vi "CRYHardware Editor.vi"() -> ()   [LabVIEW 2013]
uses:
  <vilib>/Utility/miscctls.llb/LVBoundsTypeDef.ctl
  Typedef Control/CRY6175Hardware.ctl
  CRYProject/CRYProject Editor Global.vi
  CRYWindow/SubVI/CRYMain Sub Window Global.vi
  CRYHardware Global.vi
  CRYMainGlobal.vi
  Calibration/SubVI/CRYCal Global.vi
panel:
  out "Proper VI No 2":i32 caption="Proper VI No"
  out "Hardware# Bk":T1
  in  "IN_Channel 1 Old":u16(ring) caption="Channel" items=["Mic 3/4", "Imp 1 L/R", "Imp 1 L/R Single-end", "Imp 2 L/R", "Imp 3 L/R", "Imp 4 L/R", "DUT Mic L/R", "DUT Mic DC L/R", "Cal L/R", "Input 3/4", "Output 1/2", "Output 1(-20dB)"]
  out "Hardware#":T1
  out "EndFlag":bool
  in  "AddStep":bool
  out "StepName":string
  in  "Load Test":bool caption="Load"
  out "VIMiniumBound":T2
  out "Proper VI No":i32
  in  "Board Tab":enum32{"Page 1", "Page 2"}(tab)
  in  "Cancel":bool caption="Apply"
  in  "OK":bool caption="Apply"
  in  "Main Tab":enum32{"Setting", "Help"}(tab)
  out "Microphone":bool caption="咪头"
  in  "Mic Apply":bool caption="Apply"
  in  "OUT_Impedance 2":i32(ring) caption="耳机阻抗 B" items=["1", "33"]
  in  "Mic Resis":i32 caption="咪头电阻" min=-9999 max=99999
  in  "Mic Volt":i32 caption="咪头电压" min=-999 max=9999
  in  "OUT_Impedance 1":i32(ring) caption="耳机阻抗 A" items=["1", "33 差分", "33 单端", "150", "600", "750"]
  in  "IN_Channel 2":u16(ring) caption="端口" items=["传声器 1/2", "传声器 3/4", "传声器 5/6", "传声器 7/8", "线路输入 L/R", "咪头 L/R", "耳机阻抗 B L/R", "内部校准信号 L/R"]
  out "Output":bool caption="声卡输出 1/2"
  in  "IN_Gain 2":i32(ring) caption="放大" items=["-20", "-10", "0", "10", "20", "30", "40", "50"]
  in  "OUT_Channel":u16(ring) caption="端口" items=["仿真嘴 1", "仿真嘴 2", "耳机 A/B", "耳机 A/B(L=R)"]
  out "Input 2":bool caption="声卡输入 3/4"
  in  "IN_Gain 1":i32(ring) caption="放大" items=["-20", "-10", "0", "10", "20", "30"]
  in  "IN_Channel 1":u16(ring) caption="端口" items=["传声器 3/4", "耳机阻抗 A L/R", "耳机阻抗 B L/R", "耳机阻抗 C L/R", "耳机阻抗 D L/R", "咪头电流 L/R", "咪头电压 L/R", "内部校准信号 L/R", "声卡输入 3/4", "声卡输出 1/2", "声卡输出 1(-20dB)"]
  out "Input 1":bool caption="声卡输入 1/2"
  in  "Help":string
  in  "Apply":bool
  in  "Revert":bool caption="Apply"
  in  "Save As...":bool caption="Apply"
  in  "Load...":bool caption="Apply"
  in  "stop":bool
  in  "Channel":i32=1
  in  "Hardware in":string
  in  "Calibration in":string
  # "dB"
  # "Ohm"
  # "dB"
  # "Ohm"
  # "mV"
  # "Ohm"
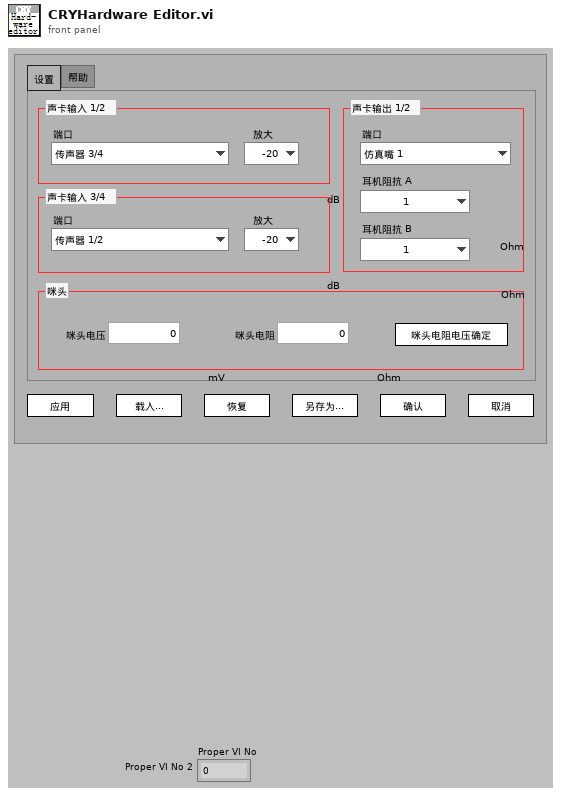
[diagram p1: front panel]
types:
  T1 = typedef "CRY6175Hardware.ctl" = cluster{"Tab Value":u16, "Help":string, "In Channel 1":u16, "In Channel 2":u16, "In Gain 1":i32, "In Gain 2":i32, "Mic Volt":i32, "Mic Resis":i32, "Out Channel":u16, "OUT_Impedance 1":u16, "OUT_Impedance 2":u16, "IN_Channel 1 Old":u16}
  T2 = typedef "LVBoundsTypeDef.ctl" = cluster{"Width":u32, "Height":u32}
  T3 = typedef "CRYStep.ctl" = cluster{"No.VI":i32, "Category":string, "StepName":string, "Seq setup flattened":string, "Comment":string, "Steps config.":bool[], "Jump config":i32[], "Start":dbl, "Increment":dbl, "Name":string, "Unit":string, "Y data":u16, "Y prefix":string, "Y dB ref":dbl, "Y unit":string, "Repeat State Array":cluster{"Start":dbl, "Increment":dbl, "Count":i32, "Num":i32}[]}
  T4 = enum16{"OK", "Yes", "YesNo", "YesNoCancel", "ReplaceAppend"}
  T5 = cluster{"Load Test":bool, "Apply":bool, "Mic Apply":bool, "OK":bool, "Cancel":bool}
  T6 = typedef "CRYData Cluster Array.ctl" = T7[]
  T7 = typedef "CRYData Cluster.ctl" = cluster{"Name":string, "Curve":cluster{"x":dbl, "y":dbl, "z":dbl}[], "X data":u16, "Y data":u16, "Z data":u16, "X axis":u16, "Y axis":u16, "Z axis":u16, "X unit":string, "Y unit":string, "Z unit":string, "X dB ref":dbl, "Y dB ref":dbl, "Z dB ref":dbl, "single val":bool, "protected":bool, "display X":bool, "display Y":bool, "display Z":bool, "Test Info":string, "Step No.":i32, "Plot Settings":cluster{"Color":u32, "Interpolation":u8, "Point Style":u8, "Line Style":u8, "Point Color":u32, "Line Width":u8, "Bar Plot Style":u8, "Fill To":i16}, "AutoProtect":bool}
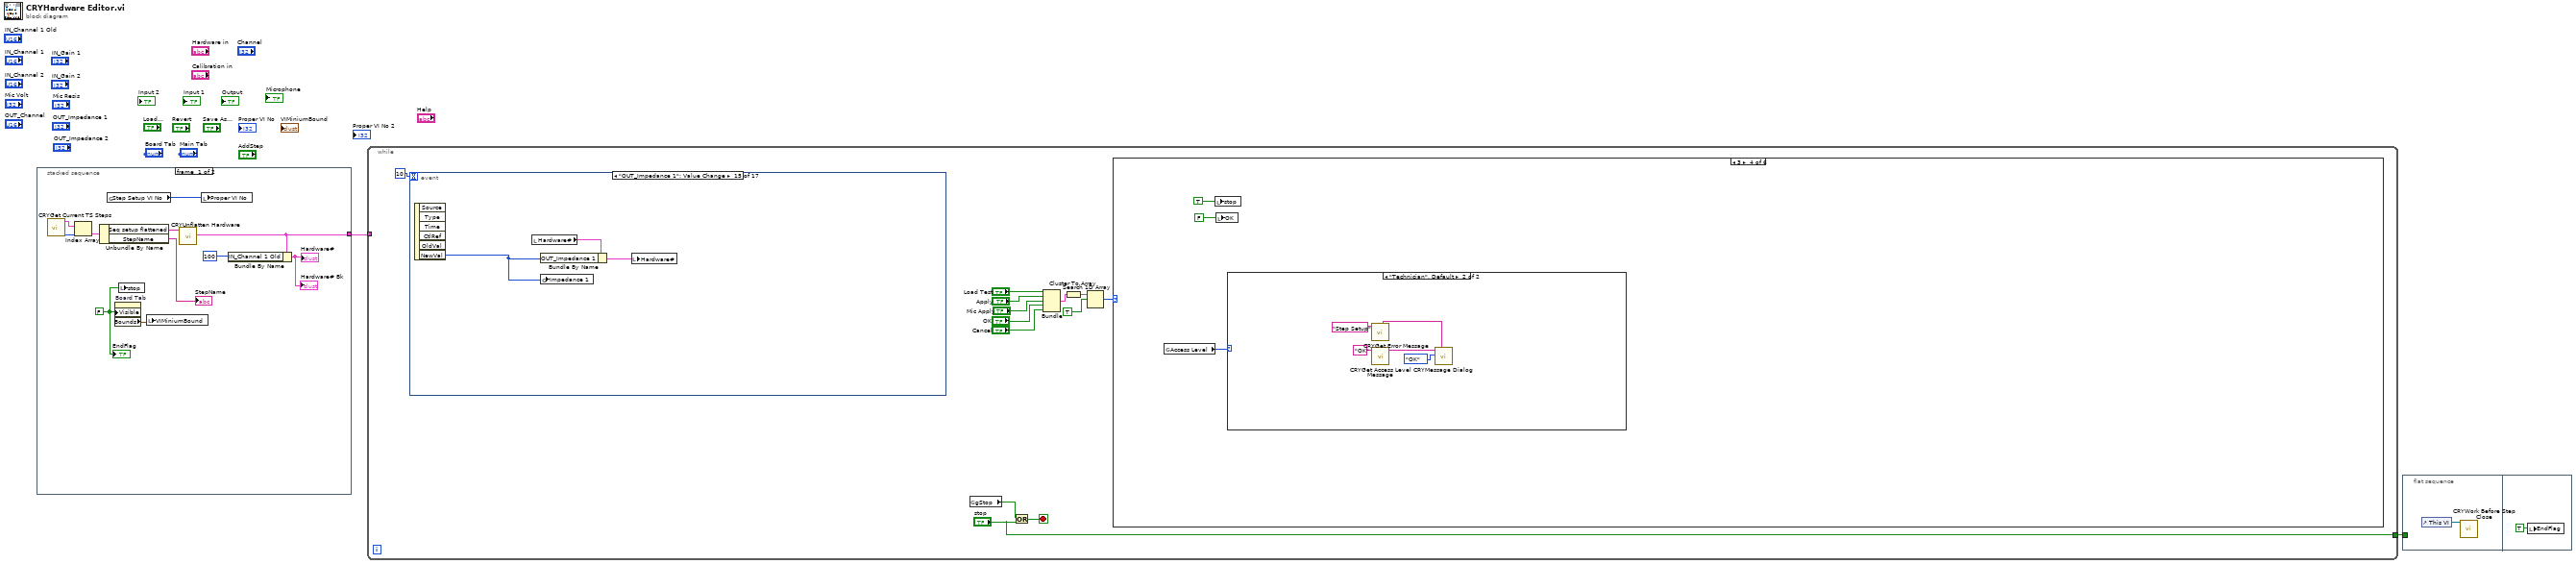
[diagram p0: block diagram]
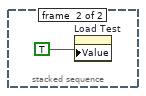
[diagram p2: hidden frame]
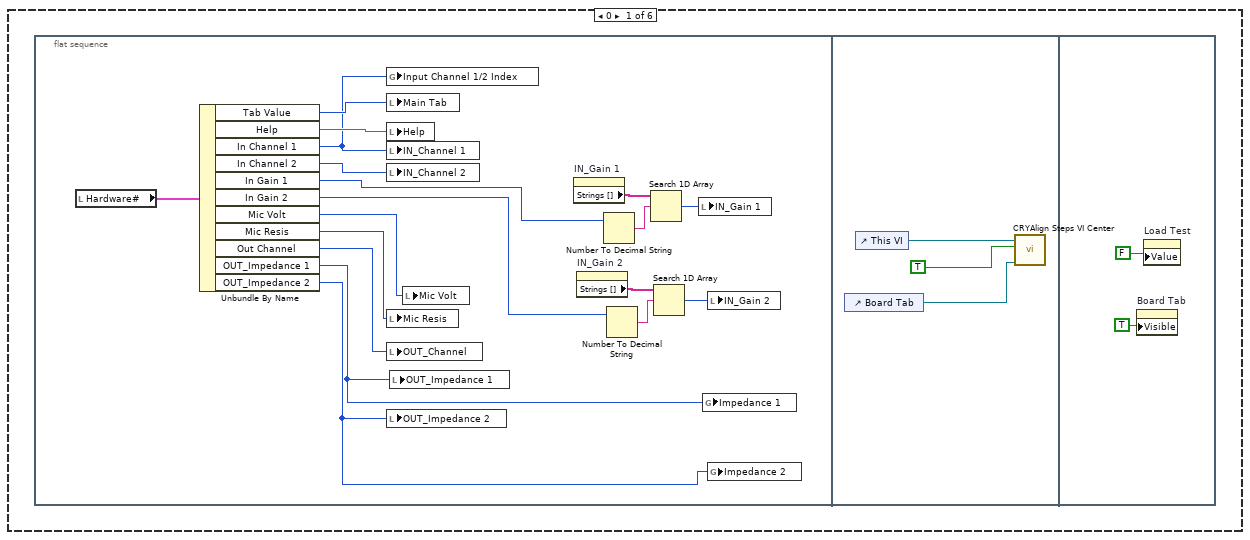
[diagram p3: hidden frame]
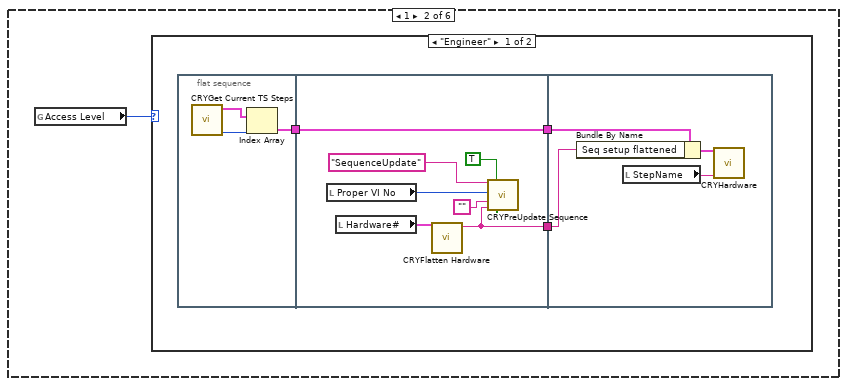
[diagram p4: hidden frame]
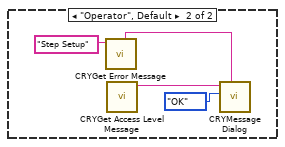
[diagram p5: hidden frame]
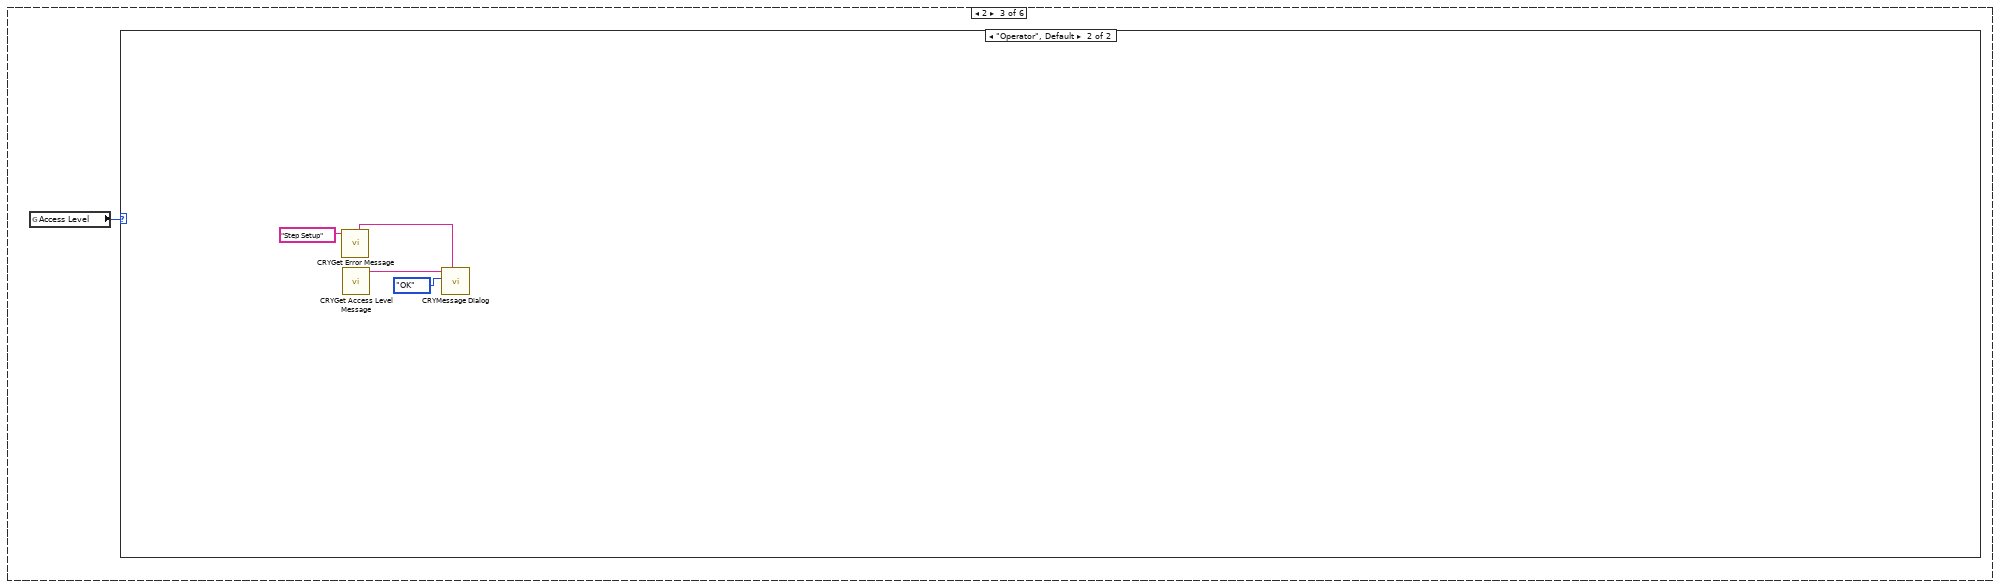
[diagram p6: hidden frame]
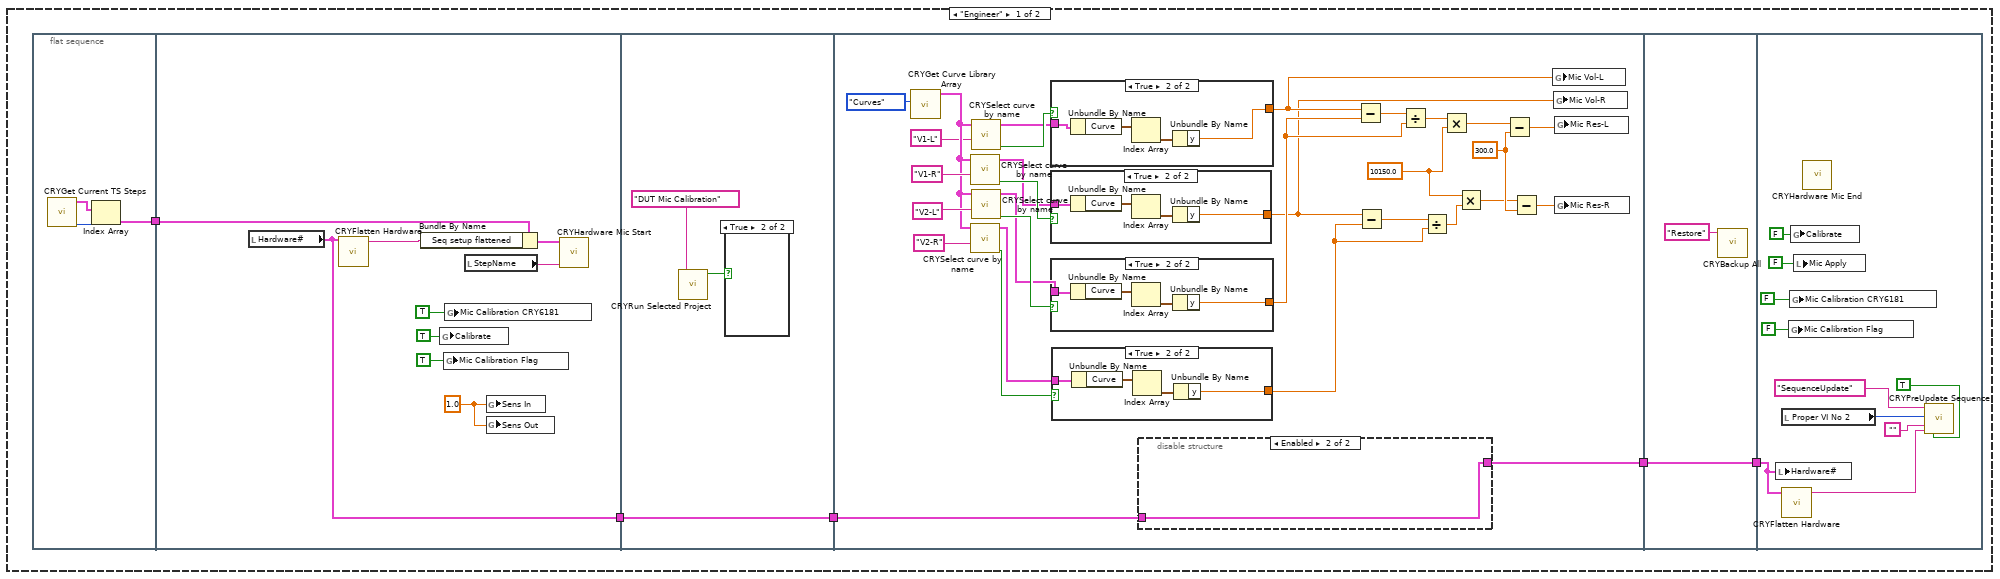
[diagram p7: hidden frame]
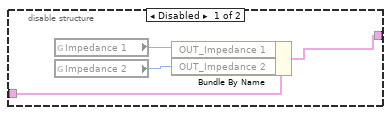
[diagram p9: hidden frame]
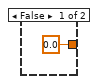
[diagram p10: hidden frame]
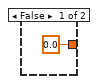
[diagram p11: hidden frame]
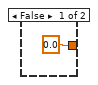
[diagram p12: hidden frame]
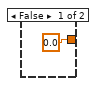
[diagram p13: hidden frame]
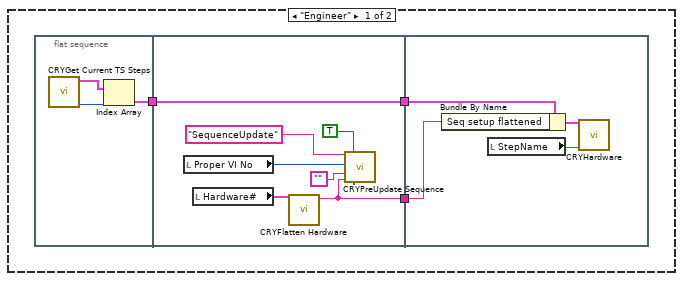
[diagram p14: hidden frame]
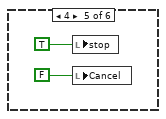
[diagram p15: hidden frame]
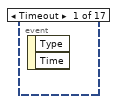
[diagram p17: hidden frame]
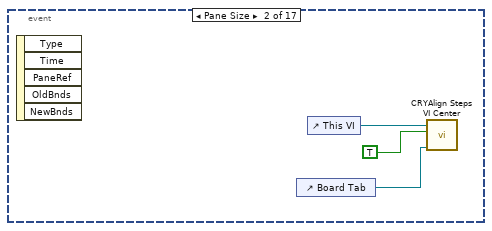
[diagram p18: hidden frame]
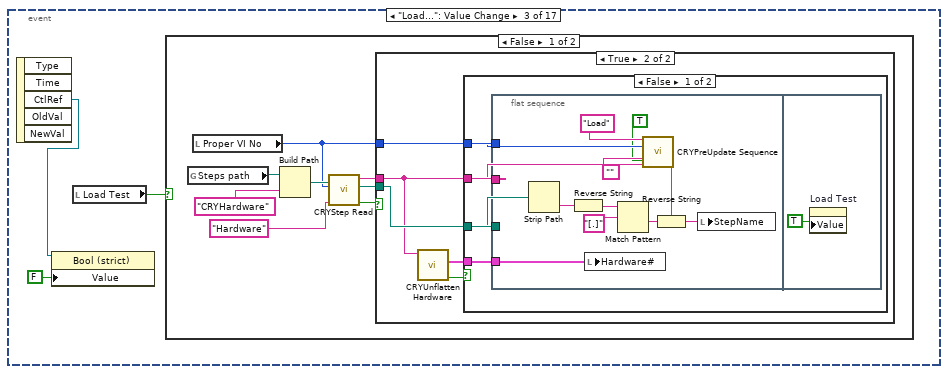
[diagram p19: hidden frame]
diagram:
  n1 = stacked-sequence {
    tunnel: [w5 _] -> w1
    frame #0 {
      w3 = FALSE ("Visible")
      n2 = call "CRYGet Current TS Steps.vi"() -> ("SelectStepNumber in Tree"=w11:i32, "Steps"=w12:T3[])  [unwired: 7 in, 3 out]
      n3 = Index Array(array=w12, index=w11) -> (element=w13:T3)
      n4 = Unbundle By Name(w13) -> ("Seq setup flattened"=w8:string, "StepName"=→"StepName":string)
      n5 = global read "CRYProject Editor Global.vi" "Step Setup VI No"() -> (w10:i32)
      n6 = property on="Board Tab" class="TabCtl (strict)"("Visible"=w3) -> ("Bounds"=w9:T2)  [unwired: 2 in, 2 out]
      n7 = local write "stop"(w3) -> ()
      n8 = local write "VIMiniumBound"(w9) -> ()
      n9 = call "CRYUnflatten Hardware.vi"("Unflatten Hardware#"=w8) -> ("Hardware"=w5:T1)  [unwired: 8 in, 2 out]
      n10 = local write "Proper VI No"(w10) -> ()
      n11 = Bundle By Name(cluster=w5, "IN_Channel 1 Old"=u16 100) -> (→"Hardware#" →"Hardware# Bk":T1)
      "EndFlag" <- w3
    }
    frame #1 {
      n12 = property on="Load Test" class="Bool (strict)"("Value"=TRUE ("Load Test")) -> ()  [unwired: 2 in, 2 out]
    }
  }
  n13 = while {
    tunnel: ["stop"] -> w2
    tunnel: w1 -> [_]
    stop <- w25 stop-if-true
    n14 = event shown="[14] \"OUT_Impedance 1\": Value Change" {
      selector: _ -> [_ _ _ _ _ _ _ _ _ _ _ _ _ _ _ _ _]
      dyn-events: _ -> [_ _ _ _ _ _ _ _ _ _ _ _ _ _ _ _ _]
      timeout: 10 -> [_ _ _ _ _ _ _ _ _ _ _ _ _ _ _ _ _]
      event Timeout {
        n15 = event-data() -> ()  [unwired: 1 in, 2 out]
      }
      event Pane Size {
        n16 = event-data() -> ()  [unwired: 1 in, 5 out]
        n17 = control-ref of="Board Tab"() -> (w192:refnum<vi>)
        n18 = control-ref of="This VI"() -> (w194:refnum<vi>)
        n19 = call "CRYAlign Steps VI Center.vi"("Tab2"=w192, "Input/Output"=TRUE, "VIRef"=w194) -> ()  [unwired: 1 in, 8 out]
      }
      event "Load...": Value Change {
        n20 = event-data() -> ("CtlRef"=w195:refnum<vi>)  [unwired: 1 in, 4 out]
        n21 = property class="Bool (strict)"(reference=w195, "Value"=FALSE) -> ()  [unwired: 1 in, 2 out]
        n22 = local read "Load Test"() -> (w197:bool)
        n23 = case shown="False" w197 {
          frame False {
            n24 = global read "CRYMainGlobal.vi" "Steps path"() -> (w204:path)
            n25 = local read "Proper VI No"() -> (w198:i32)
            n26 = Build Path(base path=w204, name or relative path="CRYHardware") -> (appended path=w205:path)
            n27 = call "CRYStep Read.vi"("Category Name"="Hardware" ("Step File Name"), "Proper VI No"=w198, "Step File Path"=w205) -> ("status"=w201:bool, "selected path"=w199:path, "Flatten Step"=w200:string)  [unwired: 1 in, 3 out]
            n28 = case shown="True" w201 {
              tunnel: w200 -> [_ w207]
              tunnel: w199 -> [_ w208]
              tunnel: w198 -> [_ w206]
              frame False {
              }
              frame True {
                n29 = call "CRYUnflatten Hardware.vi"("Unflatten Hardware#"=w207) -> ("Error?"=w210:bool, "Hardware"=w209:T1)  [unwired: 8 in, 1 out]
                n30 = case shown="False" w210 {
                  tunnel: w209 -> [w214 _]
                  tunnel: w208 -> [w213 _]
                  tunnel: w207 -> [w212 _]
                  tunnel: w206 -> [w211 _]
                  frame False {
                    n31 = flat-sequence {
                      tunnel: w214 -> [w226]
                      tunnel: w213 -> [w223]
                      tunnel: w212 -> [w222]
                      tunnel: w211 -> [w221]
                      frame #0 {
                        n32 = Strip Path(path=w223) -> (name=w216:string)  [unwired: 1 out]
                        n33 = Reverse String(1:w216) -> (0:w218:string)
                        n34 = local write "Hardware#"(w226) -> ()
                        n35 = Match Pattern(string=w218, regular expression="[.]") -> (after substring=w219:string)  [unwired: 4 out]
                        n36 = Reverse String(1:w219) -> (0:w215:string)
                        n37 = call "CRYPreUpdate Sequence.vi"("EventName"="Load", "StepName Arg3"=w215, "Proper VI No"=w221, "Project View Step Name Identifier Arg1"="", "Step flattened Arg2"=w222, "AllChangeFlg"=TRUE ("Name/Identifier")) -> ()  [unwired: 10 in]
                        n38 = local write "StepName"(w215) -> ()
                      }
                      frame #1 {
                        n39 = property on="Load Test" class="Bool (strict)"("Value"=TRUE ("Load Test")) -> ()  [unwired: 2 in, 2 out]
                      }
                    }
                  }
                  frame True {
                  }
                }
              }
            }
          }
          frame True {
          }
        }
      }
      event "Save As...": Value Change {
        w236 = "Hardware" ("Step File Name")
        n40 = event-data() -> ("CtlRef"=w228:refnum<vi>)  [unwired: 1 in, 4 out]
        n41 = local read "Hardware#"() -> (w231:T1)
        n42 = property class="Bool (strict)"(reference=w228, "Value"=FALSE) -> ()  [unwired: 1 in, 2 out]
        n43 = global read "CRYMainGlobal.vi" "Steps path"() -> (w242:path)
        n44 = call "CRYFlatten Hardware.vi"("Hardware#"=w231) -> ("Hardware# flattened"=w235:string)  [unwired: 10 in]
        n45 = Build Path(base path=w242, name or relative path="CRYHardware") -> (appended path=w238:path)
        n46 = local read "Proper VI No"() -> (w237:i32)
        n47 = call "CRYStep Write.vi"("StepIdentifier"="", "Default"=FALSE, "Proper VI No"=w237, "Category Name"=w236, "Step File Path"=w238, "Step flattened"=w235, "Step File Name"=w236) -> ("name"=w233:string, "Cancel"=w234:bool)  [unwired: 1 in, 2 out]
        n48 = Match Pattern(string=w233, regular expression=".har") -> (before substring=w230:string)  [unwired: 1 in, 3 out]
        n49 = case shown="False" w234 {
          tunnel: w230 -> [w243 _]
          frame False {
            n50 = Current VI's Path() -> (path=w244:path)
            n51 = call "CRYTitle bar update.vi"("Step name"=w243, "Editor VI path"=w244) -> ()  [unwired: 10 in]
          }
          frame True {
          }
        }
      }
      event "Revert": Value Change {
        n52 = event-data() -> ("CtlRef"=w246:refnum<vi>)  [unwired: 1 in, 4 out]
        n53 = flat-sequence {
          frame #0 {
            n54 = local read "Hardware# Bk"() -> (w247:T1)
            n55 = local write "Hardware#"(w247) -> ()
          }
          frame #1 {
            n56 = property on="Load Test" class="Bool (strict)"("Value"=TRUE ("Load Test")) -> ()  [unwired: 2 in, 2 out]
          }
        }
        n57 = property class="Bool (strict)"(reference=w246, "Value"=FALSE) -> ()  [unwired: 1 in, 2 out]
      }
      event Panel Close {
        n58 = event-data() -> ()  [unwired: 1 in, 4 out]
        n59 = control-ref of="This VI"() -> (w250:refnum<vi>)
        n60 = local write "Cancel"(TRUE ("Cancel")) -> ()
        n61 = call "CRYWork Before Step Close.vi"("StepVI Ref"=w250) -> ()  [unwired: 11 in]
      }
      event "Main Tab": Value Change {
        n62 = event-data() -> ("NewVal"=w252:enum32{"Setting", "Help"})  [unwired: 1 in, 4 out]
        n63 = local read "Hardware#"() -> (w253:T1)
        n64 = Bundle By Name(cluster=w253, "Tab Value"=w252) -> (w251:T1)
        n65 = local write "Hardware#"(w251) -> ()
      }
      event "IN_Channel 1": Value Change {
        n66 = event-data() -> ("OldVal"=w255:u16, "NewVal"=w254:u16)  [unwired: 1 in, 4 out]
        n67 = local read "Hardware#"() -> (w257:T1)
        n68 = local write "IN_Channel 1 Old"(w255) -> ()
        n69 = Bundle By Name(cluster=w257, "In Channel 1"=w254) -> (w256:T1)
        n70 = global write "CRYHardware Global.vi" "Input Channel 1/2 Index"(w254) -> ()
        n71 = local write "Hardware#"(w256) -> ()
      }
      event "IN_Gain 1": Value Change {
        n72 = event-data() -> ("NewVal"=w259:i32)  [unwired: 1 in, 5 out]
        n73 = property on="IN_Gain 1" class="Ring (strict)"() -> ("Strings []"=w261:string[])  [unwired: 2 in, 2 out]
        n74 = Index Array(array=w261, index=w259) -> (element=w260:string)
        n75 = Decimal String To Number(string=w260) -> (number=w258:i32)  [unwired: 2 in, 1 out]
        n76 = local read "Hardware#"() -> (w263:T1)
        n77 = Bundle By Name(cluster=w263, "In Gain 1"=w258) -> (w262:T1)
        n78 = local write "Hardware#"(w262) -> ()
      }
      event "IN_Channel 2": Value Change {
        n79 = event-data() -> ("NewVal"=w264:u16)  [unwired: 1 in, 5 out]
        n80 = local read "Hardware#"() -> (w266:T1)
        n81 = Bundle By Name(cluster=w266, "In Channel 2"=w264) -> (w265:T1)
        n82 = local write "Hardware#"(w265) -> ()
      }
      event "IN_Gain 2": Value Change {
        n83 = event-data() -> ("NewVal"=w268:i32)  [unwired: 1 in, 5 out]
        n84 = property on="IN_Gain 2" class="Ring (strict)"() -> ("Strings []"=w269:string[])  [unwired: 2 in, 2 out]
        n85 = Index Array(array=w269, index=w268) -> (element=w270:string)
        n86 = Decimal String To Number(string=w270) -> (number=w267:i32)  [unwired: 2 in, 1 out]
        n87 = local read "Hardware#"() -> (w272:T1)
        n88 = Bundle By Name(cluster=w272, "In Gain 2"=w267) -> (w271:T1)
        n89 = local write "Hardware#"(w271) -> ()
      }
      event "Mic Volt": Value Change {
        n90 = event-data() -> ("NewVal"=w273:i32)  [unwired: 1 in, 5 out]
        n91 = local read "Hardware#"() -> (w275:T1)
        n92 = Bundle By Name(cluster=w275, "Mic Volt"=w273) -> (w274:T1)
        n93 = local write "Hardware#"(w274) -> ()
      }
      event "Mic Resis": Value Change {
        n94 = event-data() -> ("NewVal"=w276:i32)  [unwired: 1 in, 5 out]
        n95 = local read "Hardware#"() -> (w278:T1)
        n96 = Bundle By Name(cluster=w278, "Mic Resis"=w276) -> (w277:T1)
        n97 = local write "Hardware#"(w277) -> ()
      }
      event "OUT_Channel": Value Change {
        n98 = event-data() -> ("NewVal"=w279:u16)  [unwired: 1 in, 5 out]
        n99 = local read "Hardware#"() -> (w281:T1)
        n100 = Bundle By Name(cluster=w281, "Out Channel"=w279) -> (w280:T1)
        n101 = local write "Hardware#"(w280) -> ()
      }
      event "OUT_Impedance 1": Value Change {
        n102 = event-data() -> ("NewVal"=w282:i32)  [unwired: 1 in, 5 out]
        n103 = local read "Hardware#"() -> (w284:T1)
        n104 = Bundle By Name(cluster=w284, "OUT_Impedance 1"=w282) -> (w283:T1)
        n105 = global write "CRYHardware Global.vi" "Impedance 1"(w282) -> ()
        n106 = local write "Hardware#"(w283) -> ()
      }
      event "OUT_Impedance 2": Value Change {
        n107 = event-data() -> ("NewVal"=w285:i32)  [unwired: 1 in, 5 out]
        n108 = local read "Hardware#"() -> (w287:T1)
        n109 = global write "CRYHardware Global.vi" "Impedance 2"(w285) -> ()
        n110 = Bundle By Name(cluster=w287, "OUT_Impedance 2"=w285) -> (w286:T1)
        n111 = local write "Hardware#"(w286) -> ()
      }
      event "Help": Value Change {
        n112 = event-data() -> ("NewVal"=w289:string)  [unwired: 1 in, 4 out]
        n113 = local read "Hardware#"() -> (w290:T1)
        n114 = Bundle By Name(cluster=w290, "Help"=w289) -> (w288:T1)
        n115 = local write "Hardware#"(w288) -> ()
      }
    }
    n116 = global read "CRYMain Sub Window Global.vi" "gStop"() -> (w26:bool)
    n117 = Or(x=w26, y="stop") -> (x .or. y?=w25:bool)
    n118 = Bundle("Load Test"="Load Test", "Apply"="Apply", "Mic Apply"="Mic Apply", "OK"="OK", "Cancel"="Cancel") -> (w24:T5)  [unwired: 1 out]
    n119 = Cluster To Array(cluster=w24) -> (array=w23:bool[])
    n120 = Search 1D Array(1D array=w23, element=TRUE) -> (index of element=w20:i32)  [unwired: 1 out]
    n121 = case shown="3" w20 {
      frame 0 {
        n122 = flat-sequence {
          frame #0 {
            n123 = local read "Hardware#"() -> (w45:T1)
            n124 = Unbundle By Name(w45) -> ("Tab Value"=w44:u16, "Help"=w43:string, "In Channel 1"=w29:u16, "In Channel 2"=w42:u16, "In Gain 1"=w39:i32, "In Gain 2"=w33:i32, "Mic Volt"=w41:i32, "Mic Resis"=w31:i32, "Out Channel"=w40:u16, "OUT_Impedance 1"=w30:u16, "OUT_Impedance 2"=w28:u16)
            n125 = global write "CRYHardware Global.vi" "Input Channel 1/2 Index"(w29) -> ()
            n126 = local write "Main Tab"(w44) -> ()
            n127 = local write "Help"(w43) -> ()
            n128 = local write "IN_Channel 1"(w29) -> ()
            n129 = local write "IN_Channel 2"(w42) -> ()
            n130 = local write "Mic Resis"(w31) -> ()
            n131 = local write "OUT_Channel"(w40) -> ()
            n132 = local write "OUT_Impedance 2"(w28) -> ()
            n133 = local write "OUT_Impedance 1"(w30) -> ()
            n134 = local write "Mic Volt"(w41) -> ()
            n135 = property on="IN_Gain 1" class="Ring (strict)"() -> ("Strings []"=w37:string[])  [unwired: 2 in, 2 out]
            n136 = property on="IN_Gain 2" class="Ring (strict)"() -> ("Strings []"=w35:string[])  [unwired: 2 in, 2 out]
            n137 = Number To Decimal String(number=w39) -> (decimal integer string=w38:string)  [unwired: 1 in]
            n138 = Number To Decimal String(number=w33) -> (decimal integer string=w34:string)  [unwired: 1 in]
            n139 = Search 1D Array(1D array=w37, element=w38) -> (index of element=w36:i32)  [unwired: 1 in]
            n140 = Search 1D Array(1D array=w35, element=w34) -> (index of element=w32:i32)  [unwired: 1 in]
            n141 = local write "IN_Gain 1"(w36) -> ()
            n142 = global write "CRYHardware Global.vi" "Impedance 1"(w30) -> ()
            n143 = local write "IN_Gain 2"(w32) -> ()
            n144 = global write "CRYHardware Global.vi" "Impedance 2"(w28) -> ()
          }
          frame #1 {
            n145 = control-ref of="Board Tab"() -> (w46:refnum<vi>)
            n146 = control-ref of="This VI"() -> (w48:refnum<vi>)
            n147 = call "CRYAlign Steps VI Center.vi"("Tab2"=w46, "Input/Output"=TRUE, "VIRef"=w48) -> ()  [unwired: 1 in, 8 out]
          }
          frame #2 {
            n148 = property on="Board Tab" class="TabCtl (strict)"("Visible"=TRUE) -> ()  [unwired: 2 in, 2 out]
            n149 = property on="Load Test" class="Bool (strict)"("Value"=FALSE ("Load Test")) -> ()  [unwired: 2 in, 2 out]
          }
        }
      }
      frame 1 {
        n150 = global read "CRYMainGlobal.vi" "Access Level"() -> (w51:enum16{"Engineer", "Technician", "Operator"})
        n151 = case shown="\"Engineer\"" w51 {
          frame "Engineer" {
            n152 = flat-sequence {
              tunnel: [w55] -> w53
              tunnel: [w59] -> w54
              tunnel: w53 -> [w59]
              tunnel: [w58] -> w52
              tunnel: w54 -> [w68]
              tunnel: w52 -> [w67]
              frame #0 {
                n153 = call "CRYGet Current TS Steps.vi"() -> ("SelectStepNumber in Tree"=w56:i32, "Steps"=w57:T3[])  [unwired: 1 in, 9 out]
                n154 = Index Array(array=w57, index=w56) -> (element=w55:T3)
              }
              frame #1 {
                n155 = local read "Proper VI No"() -> (w62:i32)
                n156 = local read "Hardware#"() -> (w60:T1)
                n157 = call "CRYFlatten Hardware.vi"("Hardware#"=w60) -> ("Hardware# flattened"=w58:string)  [unwired: 10 in]
                n158 = call "CRYPreUpdate Sequence.vi"("EventName"="SequenceUpdate", "Proper VI No"=w62, "Project View Step Name Identifier Arg1"="", "Step flattened Arg2"=w58, "AllChangeFlg"=TRUE ("Name/Identifier")) -> ()  [unwired: 11 in]
              }
              frame #2 {
                n159 = Bundle By Name(cluster=w68, "Seq setup flattened"=w67) -> (w66:T3)
                n160 = local read "StepName"() -> (w65:string)
                n161 = call "CRYHardware.vi"("Setup in"=w66, "Step name"=w65) -> ()  [unwired: 9 in, 5 out]
              }
            }
          }
          frame "Operator", Default {
            n162 = call "CRYGet Error Message.vi"("Kind"="Step Setup") -> ("Window Title"=w71:string)  [unwired: 5 in, 5 out]
            n163 = call "CRYGet Access Level Message.vi"() -> ("Multibyte string"=w69:string)  [unwired: 11 in]
            n164 = call "CRYMessage Dialog.vi"("Window Title"=w71, "YesNoCancel"=T4."OK", "Message Content"=w69) -> ()  [unwired: 7 in, 2 out]
          }
        }
      }
      frame 2 {
        n165 = global read "CRYMainGlobal.vi" "Access Level"() -> (w73:enum16{"Engineer", "Technician", "Operator"})
        n166 = case shown="\"Operator\", Default" w73 {
          frame "Engineer" {
            n167 = flat-sequence {
              tunnel: [w79] -> w78
              tunnel: [w82] -> w76
              tunnel: w78 -> [w90]
              tunnel: [w91] -> w77
              tunnel: w76 -> [w91]
              tunnel: w77 -> [w95]
              tunnel: [w94] -> w74
              tunnel: [w149] -> w75
              tunnel: w74 -> [w149]
              tunnel: w75 -> [w156]
              frame #0 {
                n168 = call "CRYGet Current TS Steps.vi"() -> ("SelectStepNumber in Tree"=w80:i32, "Steps"=w81:T3[])  [unwired: 1 in, 9 out]
                n169 = Index Array(array=w81, index=w80) -> (element=w79:T3)
              }
              frame #1 {
                w83 = 1.0 ("Sens In")
                n170 = local read "Hardware#"() -> (w82:T1)
                n171 = call "CRYFlatten Hardware.vi"("Hardware#"=w82) -> ("Hardware# flattened"=w89:string)  [unwired: 10 in]
                n172 = Bundle By Name(cluster=w90, "Seq setup flattened"=w89) -> (w88:T3)
                n173 = global write "CRYCal Global.vi" "Calibrate"(TRUE ("Calibrate")) -> ()
                n174 = global write "CRYHardware Global.vi" "Mic Calibration Flag"(TRUE ("Mic Calibration Flag")) -> ()
                n175 = global write "CRYCal Global.vi" "Mic Calibration CRY6181"(TRUE ("Audio Interface Calibrate")) -> ()
                n176 = local read "StepName"() -> (w87:string)
                n177 = global write "CRYCal Global.vi" "Sens In"(w83) -> ()
                n178 = global write "CRYCal Global.vi" "Sens Out"(w83) -> ()
                n179 = call "CRYHardware Mic Start.vi"("Setup in"=w88, "Step name"=w87) -> ()  [unwired: 9 in, 5 out]
              }
              frame #2 {
                n180 = call "CRYRun Selected Project.vi"("sequence name"="DUT Mic Calibration" ("y")) -> ("run state"=w93:bool)  [unwired: 10 out]
                n181 = case shown="True" w93 {
                  frame False {
                  }
                  frame True {
                  }
                }
              }
              frame #3 {
                w123 = 300.0 ("y")
                w96 = 10150.0 ("y")
                n182 = call "CRYGet Curve Library Array.vi"("Type In"=enum16{"Curves", "Values", "Results", "WFM"}."Curves") -> ("Curve/Value array"=w109:T6)  [unwired: 8 in, 2 out]
                n183 = call "CRYSelect curve by name.vi"("Curve name desired (just name, if flat data not wired)"="V1-R", "Data array"=w109) -> ("Exists?"=w106:bool, "Desired Curve"=w103:T7)  [unwired: 1 in, 7 out]
                n184 = call "CRYSelect curve by name.vi"("Curve name desired (just name, if flat data not wired)"="V2-R", "Data array"=w109) -> ("Exists?"=w108:bool, "Desired Curve"=w105:T7)  [unwired: 1 in, 7 out]
                n185 = call "CRYSelect curve by name.vi"("Curve name desired (just name, if flat data not wired)"="V1-L", "Data array"=w109) -> ("Exists?"=w113:bool, "Desired Curve"=w102:T7)  [unwired: 1 in, 7 out]
                n186 = call "CRYSelect curve by name.vi"("Curve name desired (just name, if flat data not wired)"="V2-L", "Data array"=w109) -> ("Exists?"=w107:bool, "Desired Curve"=w104:T7)  [unwired: 1 in, 7 out]
                n187 = case shown="True" w113 {
                  tunnel: w102 -> [_ w148]
                  tunnel: [0.0 ("y") w145] -> w99
                  frame False {
                  }
                  frame True {
                    n188 = Unbundle By Name(w148) -> ("Curve"=w147:cluster{"x":dbl, "y":dbl, "z":dbl}[])
                    n189 = Index Array(array=w147) -> (element=w146:cluster{"x":dbl, "y":dbl, "z":dbl})  [unwired: 1 in]
                    n190 = Unbundle By Name(w146) -> ("y"=w145:dbl)
                  }
                }
                n191 = case shown="True" w106 {
                  tunnel: w103 -> [_ w143]
                  tunnel: [0.0 ("y") w140] -> w98
                  frame False {
                  }
                  frame True {
                    n192 = Unbundle By Name(w143) -> ("Curve"=w142:cluster{"x":dbl, "y":dbl, "z":dbl}[])
                    n193 = Index Array(array=w142) -> (element=w141:cluster{"x":dbl, "y":dbl, "z":dbl})  [unwired: 1 in]
                    n194 = Unbundle By Name(w141) -> ("y"=w140:dbl)
                  }
                }
                n195 = case shown="True" w107 {
                  tunnel: w104 -> [_ w138]
                  tunnel: [0.0 ("y") w135] -> w115
                  frame False {
                  }
                  frame True {
                    n196 = Unbundle By Name(w138) -> ("Curve"=w137:cluster{"x":dbl, "y":dbl, "z":dbl}[])
                    n197 = Index Array(array=w137) -> (element=w136:cluster{"x":dbl, "y":dbl, "z":dbl})  [unwired: 1 in]
                    n198 = Unbundle By Name(w136) -> ("y"=w135:dbl)
                  }
                }
                n199 = case shown="True" w108 {
                  tunnel: w105 -> [_ w133]
                  tunnel: [0.0 ("y") w130] -> w120
                  frame False {
                  }
                  frame True {
                    n200 = Unbundle By Name(w133) -> ("Curve"=w132:cluster{"x":dbl, "y":dbl, "z":dbl}[])
                    n201 = Index Array(array=w132) -> (element=w131:cluster{"x":dbl, "y":dbl, "z":dbl})  [unwired: 1 in]
                    n202 = Unbundle By Name(w131) -> ("y"=w130:dbl)
                  }
                }
                n203 = disable-structure shown="Enabled" {
                  disable-tunnel: w95 -> [w125 w128]
                  disable-tunnel: [w124 w128] -> w94
                  frame Disabled {
                    n204 = global read "CRYHardware Global.vi" "Impedance 1"() -> (w126:i32)
                    n205 = global read "CRYHardware Global.vi" "Impedance 2"() -> (w127:i32)
                    n206 = Bundle By Name(cluster=w125, "OUT_Impedance 1"=w126, "OUT_Impedance 2"=w127) -> (w124:T1)
                  }
                  frame Enabled {
                  }
                }
                n207 = Subtract(x=w99, y=w115) -> (x-y=w114:dbl)
                n208 = Subtract(x=w98, y=w120) -> (x-y=w119:dbl)
                n209 = Divide(x=w114, y=w115) -> (x/y=w97:dbl)
                n210 = Divide(x=w119, y=w120) -> (x/y=w118:dbl)
                n211 = Multiply(x=w97, y=w96) -> (x*y=w116:dbl)
                n212 = Multiply(x=w96, y=w118) -> (x*y=w117:dbl)
                n213 = Subtract(x=w116, y=w123) -> (x-y=w121:dbl)
                n214 = Subtract(x=w117, y=w123) -> (x-y=w122:dbl)
                n215 = global write "CRYHardware Global.vi" "Mic Vol-L"(w99) -> ()
                n216 = global write "CRYHardware Global.vi" "Mic Vol-R"(w98) -> ()
                n217 = global write "CRYHardware Global.vi" "Mic Res-L"(w121) -> ()
                n218 = global write "CRYHardware Global.vi" "Mic Res-R"(w122) -> ()
              }
              frame #4 {
                n219 = call "CRYBackup All.vi"("sOption"="Restore") -> ()  [unwired: 11 in]
              }
              frame #5 {
                n220 = local write "Hardware#"(w156) -> ()
                n221 = local read "Proper VI No 2"() -> (w155:i32)
                n222 = call "CRYFlatten Hardware.vi"("Hardware#"=w156) -> ("Hardware# flattened"=w151:string)  [unwired: 10 in]
                n223 = global write "CRYHardware Global.vi" "Mic Calibration Flag"(FALSE ("Mic Calibration Flag")) -> ()
                n224 = global write "CRYCal Global.vi" "Mic Calibration CRY6181"(FALSE ("Audio Interface Calibrate")) -> ()
                n225 = global write "CRYCal Global.vi" "Calibrate"(FALSE ("Calibrate")) -> ()
                n226 = local write "Mic Apply"(FALSE ("Mic Apply")) -> ()
                n227 = call "CRYHardware Mic End.vi"() -> ()  [unwired: 16 in]
                n228 = call "CRYPreUpdate Sequence.vi"("EventName"="SequenceUpdate", "Proper VI No"=w155, "Project View Step Name Identifier Arg1"="", "Step flattened Arg2"=w151, "AllChangeFlg"=TRUE ("Name/Identifier")) -> ()  [unwired: 11 in]
              }
            }
          }
          frame "Operator", Default {
            n229 = call "CRYGet Error Message.vi"("Kind"="Step Setup") -> ("Window Title"=w163:string)  [unwired: 5 in, 5 out]
            n230 = call "CRYGet Access Level Message.vi"() -> ("Multibyte string"=w161:string)  [unwired: 11 in]
            n231 = call "CRYMessage Dialog.vi"("Window Title"=w163, "YesNoCancel"=T4."OK", "Message Content"=w161) -> ()  [unwired: 7 in, 2 out]
          }
        }
      }
      frame 3 {
        n232 = global read "CRYMainGlobal.vi" "Access Level"() -> (w165:enum16{"Engineer", "Technician", "Operator"})
        n233 = local write "stop"(TRUE ("stop")) -> ()
        n234 = local write "OK"(FALSE ("OK")) -> ()
        n235 = case shown="\"Technician\", Default" w165 {
          frame "Engineer" {
            n236 = flat-sequence {
              tunnel: [w171] -> w170
              tunnel: [w175] -> w169
              tunnel: w170 -> [w175]
              tunnel: [w174] -> w168
              tunnel: w169 -> [w184]
              tunnel: w168 -> [w183]
              frame #0 {
                n237 = call "CRYGet Current TS Steps.vi"() -> ("SelectStepNumber in Tree"=w172:i32, "Steps"=w173:T3[])  [unwired: 1 in, 9 out]
                n238 = Index Array(array=w173, index=w172) -> (element=w171:T3)
              }
              frame #1 {
                n239 = local read "Proper VI No"() -> (w178:i32)
                n240 = local read "Hardware#"() -> (w176:T1)
                n241 = call "CRYFlatten Hardware.vi"("Hardware#"=w176) -> ("Hardware# flattened"=w174:string)  [unwired: 10 in]
                n242 = call "CRYPreUpdate Sequence.vi"("EventName"="SequenceUpdate", "Proper VI No"=w178, "Project View Step Name Identifier Arg1"="", "Step flattened Arg2"=w174, "AllChangeFlg"=TRUE ("Name/Identifier")) -> ()  [unwired: 11 in]
              }
              frame #2 {
                n243 = Bundle By Name(cluster=w184, "Seq setup flattened"=w183) -> (w182:T3)
                n244 = local read "StepName"() -> (w181:string)
                n245 = call "CRYHardware.vi"("Setup in"=w182, "Step name"=w181) -> ()  [unwired: 9 in, 5 out]
              }
            }
          }
          frame "Technician", Default {
            n246 = call "CRYGet Error Message.vi"("Kind"="Step Setup") -> ("Window Title"=w187:string)  [unwired: 5 in, 5 out]
            n247 = call "CRYGet Access Level Message.vi"("sAction"="OK") -> ("Multibyte string"=w189:string)  [unwired: 10 in]
            n248 = call "CRYMessage Dialog.vi"("Window Title"=w187, "YesNoCancel"=T4."OK", "Message Content"=w189) -> ()  [unwired: 7 in, 2 out]
          }
        }
      }
      frame 4 {
        n249 = local write "stop"(TRUE ("stop")) -> ()
        n250 = local write "Cancel"(FALSE ("Cancel")) -> ()
      }
      frame Default {
      }
    }
  }
  n251 = flat-sequence {
    tunnel: w2 -> [_]
    frame #0 {
      n252 = control-ref of="This VI"() -> (w291:refnum<vi>)
      n253 = call "CRYWork Before Step Close.vi"("StepVI Ref"=w291) -> ()  [unwired: 11 in]
    }
    frame #1 {
      n254 = local write "EndFlag"(TRUE ("EndFlag")) -> ()
    }
  }
